vi "Actor Core.vi"(8 "error in":errorcluster, 11 "ModelSynchronouslyRequestsManyDoubleFloats In":refnum<class "ModelSynchronouslyRequestsManyDoubleFloats.lvclass">) -> (0 "error out":errorcluster, 3 "Actor out":refnum<class "Actor.lvclass">)   [LabVIEW 2020, in "ModelSynchronouslyRequestsManyDoubleFloats.lvclass"]
doc: "(<B>Filename</B>: Actor Framework.lvlib:Actor.lvclass:Actor Core.vi)\n\nReceives messages to the actor, reacts to them, and initiates any error handling that may shut the actor down.\n\nDescendant classes may override this VI to append parallel tasks for the actor to complete while it handles messages. Overrides use the Call Parent Method node."
uses:
  ModelSynchronouslyRequestsManyDoubleFloats.lvclass
  ModelSynchronouslyRequestsManyDoubleFloats.lvclass/ModelSynchronouslyRequestsManyDoubleFloats.ctl
  d8256b01-5b3f-4abd-bc08-c566e1cf3068.vi
  69233fbd-ecda-40a5-8579-e87e8d509e23.vi
  f1727119-a80e-48e9-bea4-66fc80b569fd.vi
  79351e9e-a154-484d-9ac9-bef871106410.vi
  Source/IModel/IModel/IModel.lvclass
  <vilib>/ActorFramework/Actor/Actor.lvclass
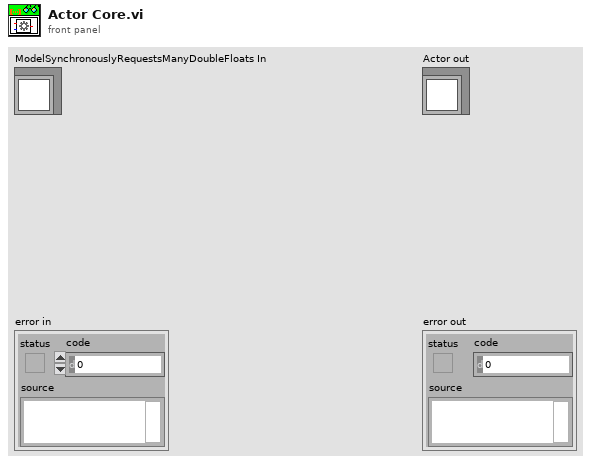
[diagram p1: front panel]
types:
  T1 = cluster{"Data":dbl, "timed out?":bool, "error out":errorcluster}
  T2 = cluster{"Data":dbl, "timed out?":bool, "error out":errorcluster}[]
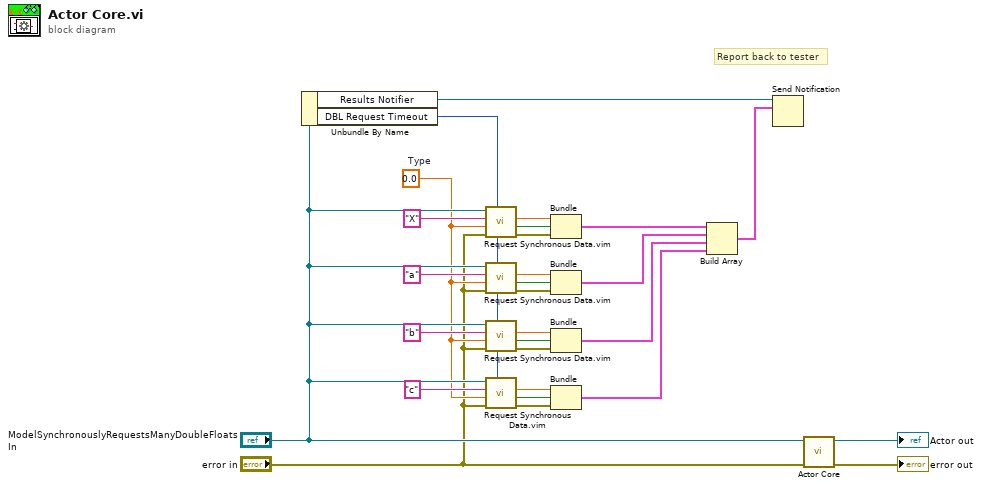
[diagram p0: block diagram]
diagram:
  w5 = 0.0  # Type
  # "Report back to tester"
  n1 = Unbundle By Name("ModelSynchronouslyRequestsManyDoubleFloats In") -> ("Results Notifier"=w21:refnum<notifier>, "DBL Request Timeout"=w1:i32)
  n2 = call "Request Synchronous Data.vim"("Timeout In ms (-1)"=w1, "error in (no error)"="error in", "Type"=w5, "Datum Name"="X", "IObserver In"="ModelSynchronouslyRequestsManyDoubleFloats In") -> ("error out"=w20:errorcluster, "timed out?"=w19:bool, "Data"=w18:dbl)  [unwired: 3 in, 1 out]
  n3 = call "Request Synchronous Data.vim"("Timeout In ms (-1)"=w1, "error in (no error)"="error in", "Type"=w5, "Datum Name"="a", "IObserver In"="ModelSynchronouslyRequestsManyDoubleFloats In") -> ("error out"=w24:errorcluster, "timed out?"=w25:bool, "Data"=w26:dbl)  [unwired: 3 in, 1 out]
  n4 = call "Request Synchronous Data.vim"("Timeout In ms (-1)"=w1, "error in (no error)"="error in", "Type"=w5, "Datum Name"="b", "IObserver In"="ModelSynchronouslyRequestsManyDoubleFloats In") -> ("error out"=w13:errorcluster, "timed out?"=w12:bool, "Data"=w11:dbl)  [unwired: 3 in, 1 out]
  n5 = call "Request Synchronous Data.vim"("Timeout In ms (-1)"=w1, "error in (no error)"="error in", "Type"=w5, "Datum Name"="c", "IObserver In"="ModelSynchronouslyRequestsManyDoubleFloats In") -> ("error out"=w8:errorcluster, "timed out?"=w9:bool, "Data"=w10:dbl)  [unwired: 3 in, 1 out]
  n6 = Bundle("Data"=w18, "timed out?"=w19, "error out"=w20) -> (w15:T1)  [unwired: 1 in]
  n7 = Bundle("Data"=w26, "timed out?"=w25, "error out"=w24) -> (w23:T1)  [unwired: 1 in]
  n8 = Bundle("Data"=w11, "timed out?"=w12, "error out"=w13) -> (w3:T1)  [unwired: 1 in]
  n9 = Bundle("Data"=w10, "timed out?"=w9, "error out"=w8) -> (w2:T1)  [unwired: 1 in]
  n10 = Build Array(w15, w23, w3, w2) -> (w22:T2)
  n11 = Send Notification(notification=w22, notifier=w21) -> ()  [unwired: 1 in, 2 out]
  n12 = call-parent "Actor Core.vi"("error in"="error in", "Actor in"="ModelSynchronouslyRequestsManyDoubleFloats In") -> ("error out"=→"error out":errorcluster, "Actor out"=→"Actor out":refnum<class "Actor.lvclass">)  [unwired: 8 in]
